vi "read parameters.vi"(8 "error in (no error)":errorcluster, 10 "refnum in":refnum<file>, 11 "Task in":refnum<class "Task.lvclass">) -> (0 "error out":errorcluster, 3 "Task out":refnum<class "Task.lvclass">)   [LabVIEW 2020, in "Tasks.lvlib" / "Task.lvclass"]
uses:
  Task.lvclass
  Task.lvclass/Task.ctl
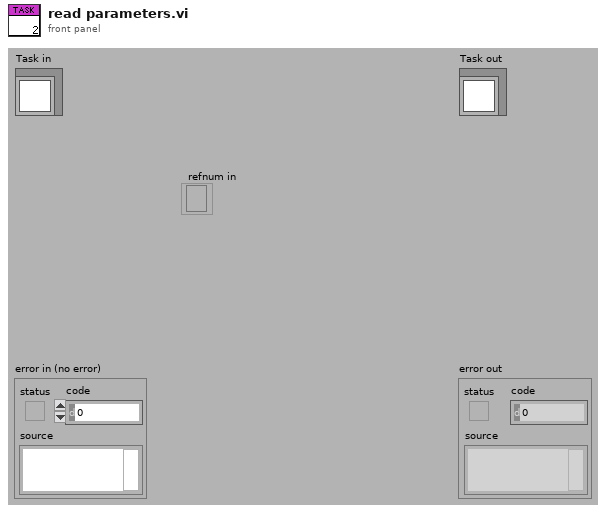
[diagram p1: front panel]
types:
  T1 = typedef "Tasks.lvlib/Task.lvclass/parameters.ctl" = cluster{"Duration (s)":dbl, "Run?":bool}
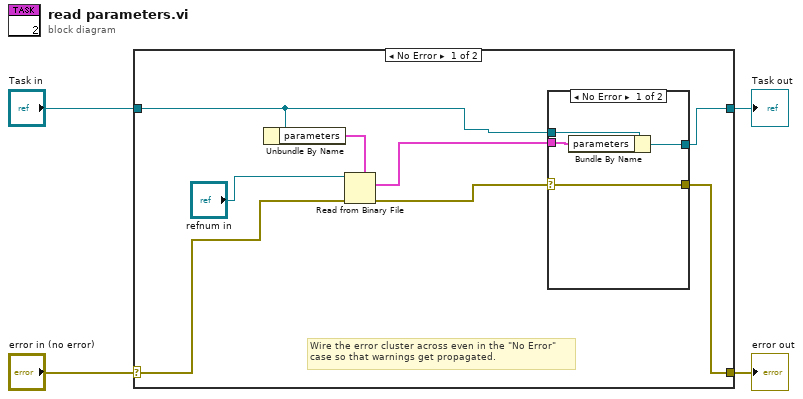
[diagram p0: block diagram]
diagram:
  n1 = case shown="No Error" "error in (no error)" {
    selector: "error in (no error)" -> [w5 w20]
    tunnel: [w9 w20] -> w3
    tunnel: [w6 w19] -> w1
    tunnel: "Task in" -> [w8 w19]
    frame No Error {
      # "Wire the error cluster across even in the \"No Error\"\ncase so that warnings get propagated."
      n2 = Unbundle By Name(w8) -> ("parameters"=w11:T1)
      n3 = Read from Binary File(5:w11, 8:w5, 11:"refnum in") -> (0:w10:errorcluster, 2:w7:T1)  [unwired: 3 in, 2 out]
      n4 = case shown="No Error" w10 {
        selector: w10 -> [w16 w18]
        tunnel: [w16 w18] -> w9
        tunnel: w8 -> [w15 w17]
        tunnel: w7 -> [w14 _]
        tunnel: [w13 w17] -> w6
        frame No Error {
          n5 = Bundle By Name(cluster=w15, "parameters"=w14) -> (w13:refnum<class "Task.lvclass">)
        }
        frame Error {
        }
      }
    }
    frame Error {
    }
  }
  "error out" <- w3
  "Task out" <- w1
